vi "MB Ethernet Slave Demon.vi"(7 "Data Reference":T1, 9 "Period":u32=100, 10 "Timeout":i32=30000, 11 "Port":u16=502) -> (2 "Demon Running":bool, 3 "# of connections":i32)   [LabVIEW 2019, in "NI_modbus_upd.lvlib"]
uses:
  NI_modbus_upd.lvlib
  Ctl/MB Ethernet Connection Function.ctl
  MB Globals.vi
panel:
  in  "Case Constant\n(See Context Help)":bool
  # "VI Name: MB Ethernet Slave Demon.vi\nPurpose: Modbus Demon\nMonitor a single port, but can accept multiple connections."
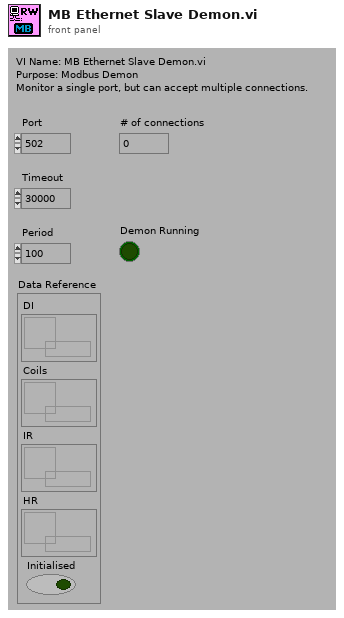
[diagram p1: front panel]
types:
  T1 = cluster{"DI":refnum<data-value>, "Coils":refnum<data-value>, "IR":refnum<data-value>, "HR":refnum<data-value>, "Initialised":bool}
  T2 = typedef "NI_modbus_upd.lvlib/MB Ethernet Connection Function.ctl" = enum16{"Init", "Add Connection", "Get All Connections", "Delete Connection"}
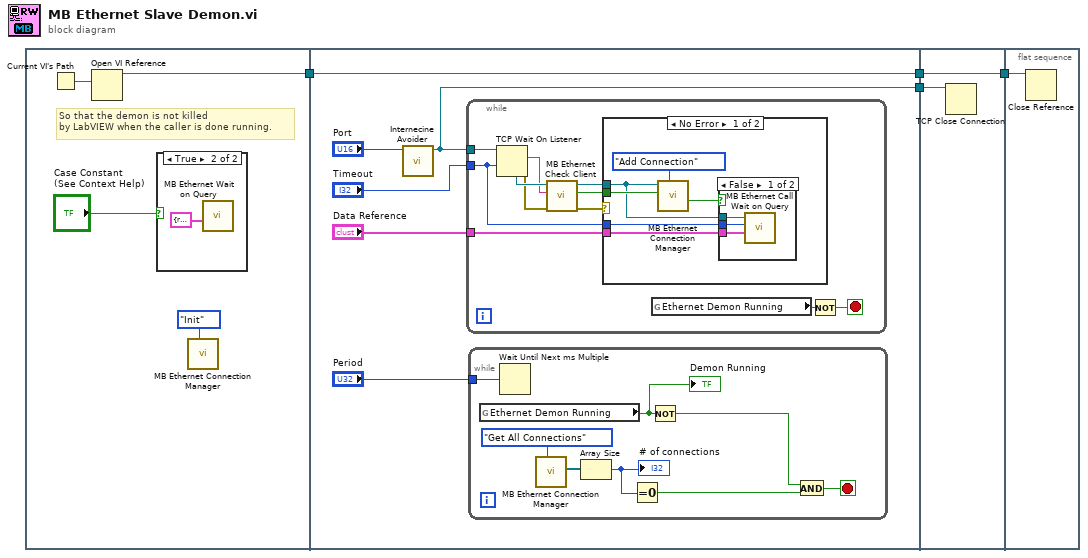
[diagram p0: block diagram]
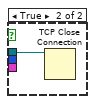
[diagram p3: hidden frame]
diagram:
  n1 = flat-sequence {
    tunnel: [w7] -> w4
    tunnel: w4 -> [w11]
    tunnel: [w11] -> w3
    tunnel: [w13] -> w2
    tunnel: [w45] -> w1
    tunnel: w2 -> [w46]
    tunnel: w3 -> [w45]
    tunnel: w1 -> [w47]
    frame #0 {
      # "So that the demon is not killed\nby LabVIEW when the caller is done running."
      n2 = Current VI's Path() -> (path=w8:path)
      n3 = Open VI Reference(vi path=w8) -> (vi reference=w7:refnum<vi>)  [unwired: 5 in, 1 out]
      n4 = case shown="True" "Case Constant\n(See Context Help)" {
        frame False {
        }
        frame True {
          n5 = call "MB Ethernet Wait on Query.vi"("Data Reference"=T1 {"DI"=refnum, "Coils"=refnum, "IR"=refnum, "HR"=refnum, "Initialised"=FALSE}) -> ()  [unwired: 11 in]
        }
      }
      n6 = call "MB Ethernet Connection Manager.vi"("Function"=MB_Ethernet_Connection_Function."Init") -> ()  [unwired: 8 in, 3 out]
    }
    frame #1 {
      n7 = call <vilib>:"Internecine Avoider.vi"("port"="Port") -> ("connection ID"=w13:refnum<k5>)  [unwired: 9 in, 1 out]
      n8 = while {
        tunnel: w13 -> [w26]
        tunnel: "Timeout" -> [w17]
        tunnel: "Data Reference" -> [w16]
        stop <- w24 stop-if-true
        n9 = TCP Wait On Listener(9:w17, 11:w26) -> (0:w21:errorcluster, 2:w19:string, 4:w23:refnum<k5>)  [unwired: 2 in, 2 out]
        n10 = call "MB Ethernet Check Client.vi"("error in (no error)"=w21, "Remote Address"=w19, "Connection ID in"=w23) -> ("error out"=w20:errorcluster, "Priority"=w18:bool, "Connection ID out"=w22:refnum<k5>)  [unwired: 6 in]
        n11 = case shown="No Error" w20 {
          tunnel: w22 -> [w28 _]
          tunnel: w18 -> [w30 _]
          tunnel: w17 -> [w29 _]
          tunnel: w16 -> [w27 _]
          frame No Error {
            n12 = call "MB Ethernet Connection Manager.vi"("Function"=MB_Ethernet_Connection_Function."Add Connection", "Priority"=w30, "Connection ID"=w28) -> ("Close Connection"=w31:bool)  [unwired: 6 in, 2 out]
            n13 = case shown="False" w31 {
              tunnel: w28 -> [w35 w36]
              tunnel: w29 -> [w34 _]
              tunnel: w27 -> [w33 _]
              frame False {
                n14 = call "MB Ethernet Call Wait on Query.vi"("Data Reference"=w33, "Timeout"=w34, "Connection ID"=w35) -> ()  [unwired: 9 in]
              }
              frame True {
                n15 = TCP Close Connection(connection ID=w36) -> ()  [unwired: 2 in, 2 out]
              }
            }
          }
          frame Error {
          }
        }
        n16 = global read "MB Globals.vi" "Ethernet Demon Running"() -> (w25:bool)
        n17 = Not(x=w25) -> (.not. x?=w24:bool)
      }
      n18 = while {
        tunnel: "Period" -> [w41]
        stop <- w38 stop-if-true
        n19 = global read "MB Globals.vi" "Ethernet Demon Running"() -> (w44:bool)
        "Demon Running" <- w44
        n20 = Wait Until Next ms Multiple(millisecond multiple=w41) -> ()  [unwired: 1 out]
        n21 = call "MB Ethernet Connection Manager.vi"("Function"=MB_Ethernet_Connection_Function."Get All Connections") -> ("Connection IDs"=w42:refnum<k5>[])  [unwired: 8 in, 2 out]
        n22 = Array Size(array=w42) -> (size(s)=w39:i32)
        "# of connections" <- w39
        n23 = Equal To 0?(x=w39) -> (x = 0?=w40:bool)
        n24 = Not(x=w44) -> (.not. x?=w37:bool)
        n25 = And(x=w37, y=w40) -> (x .and. y?=w38:bool)
      }
    }
    frame #2 {
      n26 = TCP Close Connection(connection ID=w46) -> ()  [unwired: 2 in, 2 out]
    }
    frame #3 {
      n27 = Close Reference(reference=w47) -> ()  [unwired: 1 in, 1 out]
    }
  }
